vi "BLE_Hash256.vi"(0 "Password":string, 5 "RandNumber":u8[](array[numeric]), 11 "error in (no error)":errorcluster) -> (4 "Hash256":u8[](array[numeric]) format="%.0x", 6 "Hash256":string, 15 "error out":errorcluster)   [LabVIEW 2020, in "BLE.lvlib"]
uses:
  BLE.lvlib
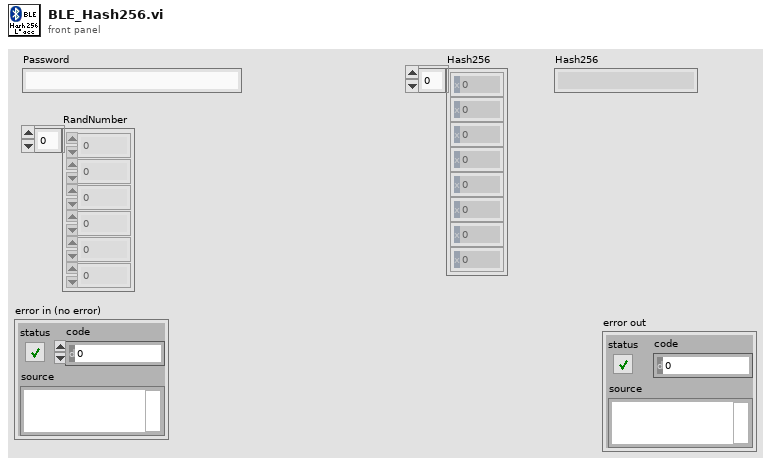
[diagram p1: front panel]
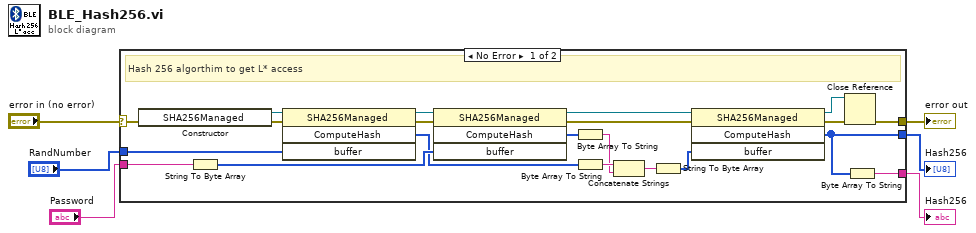
[diagram p0: block diagram]
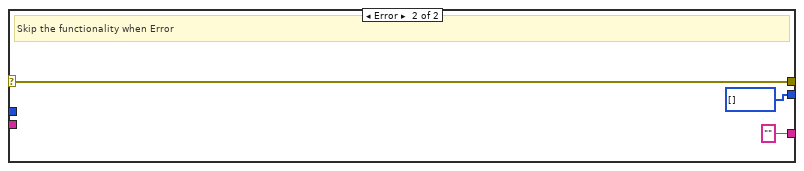
[diagram p2: hidden frame]
diagram:
  n1 = case shown="No Error" "error in (no error)" {
    selector: "error in (no error)" -> [w15 w30]
    tunnel: "Password" -> [w27 _]
    tunnel: [w25 u8[] [] ("ComputeHash")] -> w5
    tunnel: [w16 w30] -> w4
    tunnel: [w14 "" ("string")] -> w2
    tunnel: "RandNumber" -> [w7 _]
    frame No Error {
      # "Hash 256 algorthim to get L* access"
      n2 = constructor class="SHA256Managed"(error in=w15) -> (reference out=w20:refnum<k24>, error out=w19:errorcluster)  [unwired: 2 in, 1 out]
      n3 = String To Byte Array(string=w27) -> (unsigned byte array=w26:u8[])
      n4 = invoke class="SHA256Managed" method="ComputeHash"(reference=w20, error in=w19, "buffer"=w7) -> (reference out=w22:refnum<k24>, error out=w24:errorcluster, "ComputeHash"=w13:u8[])  [unwired: 1 in, 1 out]
      n5 = invoke class="SHA256Managed" method="ComputeHash"(reference=w22, error in=w24, "buffer"=w26) -> (reference out=w21:refnum<k24>, error out=w23:errorcluster, "ComputeHash"=w12:u8[])  [unwired: 1 in, 1 out]
      n6 = Byte Array To String(unsigned byte array=w12) -> (string=w10:string)
      n7 = Byte Array To String(unsigned byte array=w13) -> (string=w11:string)
      n8 = Concatenate Strings(w11, w10) -> (w9:string)
      n9 = String To Byte Array(string=w9) -> (unsigned byte array=w8:u8[])
      n10 = invoke class="SHA256Managed" method="ComputeHash"(reference=w21, error in=w23, "buffer"=w8) -> (reference out=w17:refnum<k24>, error out=w18:errorcluster, "ComputeHash"=w25:u8[])  [unwired: 1 in, 1 out]
      n11 = Close Reference(reference=w17, error in (no error)=w18) -> (error out=w16:errorcluster)
      n12 = Byte Array To String(unsigned byte array=w25) -> (string=w14:string)
    }
    frame Error {
      # "Skip the functionality when Error"
    }
  }
  "Hash256" <- w5
  "Hash256" <- w2
  "error out" <- w4
